vi "fgv_4610_return.vi"(7 "cmd":T2, 11 "output":T1 {"DC current[A]" format="%.2f"; "DC voltage[V]" format="%.1f"}) -> (3 "output 2":T1 {"DC current[A]" format="%.2f"; "DC voltage[V]" format="%.1f"})   [LabVIEW 2019]
uses:
  _ctrl/rw.ctl
  _ctrl/BP4610_return.ctl
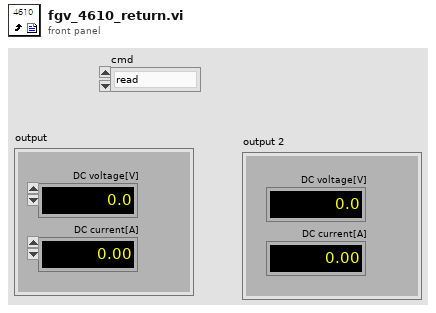
[diagram p1: front panel]
types:
  T1 = typedef "BP4610_return.ctl" = cluster{"DC voltage[V]":dbl, "DC current[A]":dbl}
  T2 = typedef "rw.ctl" = enum16{"read", "write"}
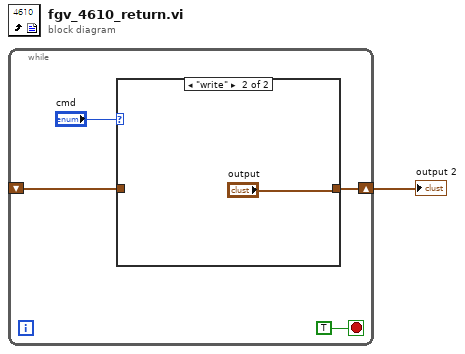
[diagram p0: block diagram]
diagram:
  n1 = while {
    shift-right: [w3] -> w1
    shift-left: _ -> [w2]
    stop <- TRUE stop-if-true
    n2 = case shown="\"write\"" "cmd" {
      tunnel: [w6 "output"] -> w3
      tunnel: w2 -> [w6 _]
      frame "read", Default {
      }
      frame "write" {
      }
    }
  }
  "output 2" <- w1
